vi "module.vi"(6 "cmd channel":T2) -> (7 "response":T2)   [LabVIEW 2023, in "Camera Calibration.lvlib"]
uses:
  Camera Calibration.lvlib
  <extravilib>/ChannelInstances/Messenger-t'Message Queue.lvlib-Message Cluster.ctl'/))Channel.ctl
  <vilib>/DLR/CMH Library/Message Queue/Message Cluster.ctl
  <vilib>/DLR/Graphs/Detail Graph/Detail Graph.lvclass
  C:/Program Files/National Instruments/LabVIEW 2023/vi.lib/DLR/Graphs/Base Graph/Base Graph.lvclass
  <vilib>/Utility/miscctls.llb/LVPoint32TypeDef.ctl
  <vilib>/DLR/CMH Library/Message Queue/Enqueue Message.vi
  c1bcd614-dbd8-4c7e-9590-75ab6b9c2f97.vi
  5a16af59-63b5-408a-9197-58993c91bf3e.vi
  e40aba5b-5f5a-4406-9bae-245098e35ac7.vi
  702dd1aa-c489-4f6b-9c67-8e13a44c3bd1.vi
  480c1a3a-5302-4998-8e9b-bb535253195f.vi
  <extravilib>/ChannelInstances/Messenger-t'Message Queue.lvlib-Message Cluster.ctl'/Write With Abort.vi
  <extravilib>/ChannelInstances/Event Messenger-bool/Instantiate.vi
  <extravilib>/ChannelInstances/Event Messenger-bool/))Channel.vi
  <extravilib>/ChannelInstances/Messenger-t'Message Queue.lvlib-Message Cluster.ctl'/Endpoint.vi
  <vilib>/Utility/inputDevices.llb/keyboardAcquire.vi
  <vilib>/Utility/error.llb/Error Cluster From Error Code.vi
  <vilib>/ErrorRing/Error Ring.xnode
  <vilib>/DLR/CMH Library/Message Queue.lvlib
  <vilib>/DLR/CMH Library/Message Queue Helper.lvlib
  <extravilib>/ChannelInstances/Event Messenger-bool.lvlib
  <vilib>/DLR/Graphs/Base Graph/Base Graph.lvclass
  OpenCV-Calibration-LabVIEW-Wrapper/build/x64/Debug/OpenCV-Calibration-LabVIEW-Wrapper.dll
  C:/Program Files/National Instruments/LabVIEW 2023/vi.lib/DLR/Graphs/Detail Graph/Detail Graph.lvclass
  <extravilib>/ChannelInstances/Messenger-t'Message Queue.lvlib-Message Cluster.ctl'.lvlib
panel:
  in  "Main Control":enum32{"Feature Extraction", "Empty"}(tab)
  out "Selection Mask":T1 {"Polygon"."Y [px]" format="%#_5g"}
  out "Extracted Points":cluster{"X [px]":sgl, "Y [px]":sgl}[](array[cluster]) {"Y [px]" format="%#_5g"; "X [px]" format="%#_5g"}
  in  "Extract Corners":bool
  out "Intensity Width Graph":cluster{"Array":dbl[], "Array":dbl[]}(graph)
  out "Signal Map":u16[][](graph)
  out "Intensity Height Graph":cluster{"Array":dbl[], "Array":dbl[]}(graph)
  in  "Image #":u16
  in  "Close Button":bool
  out "Log":string
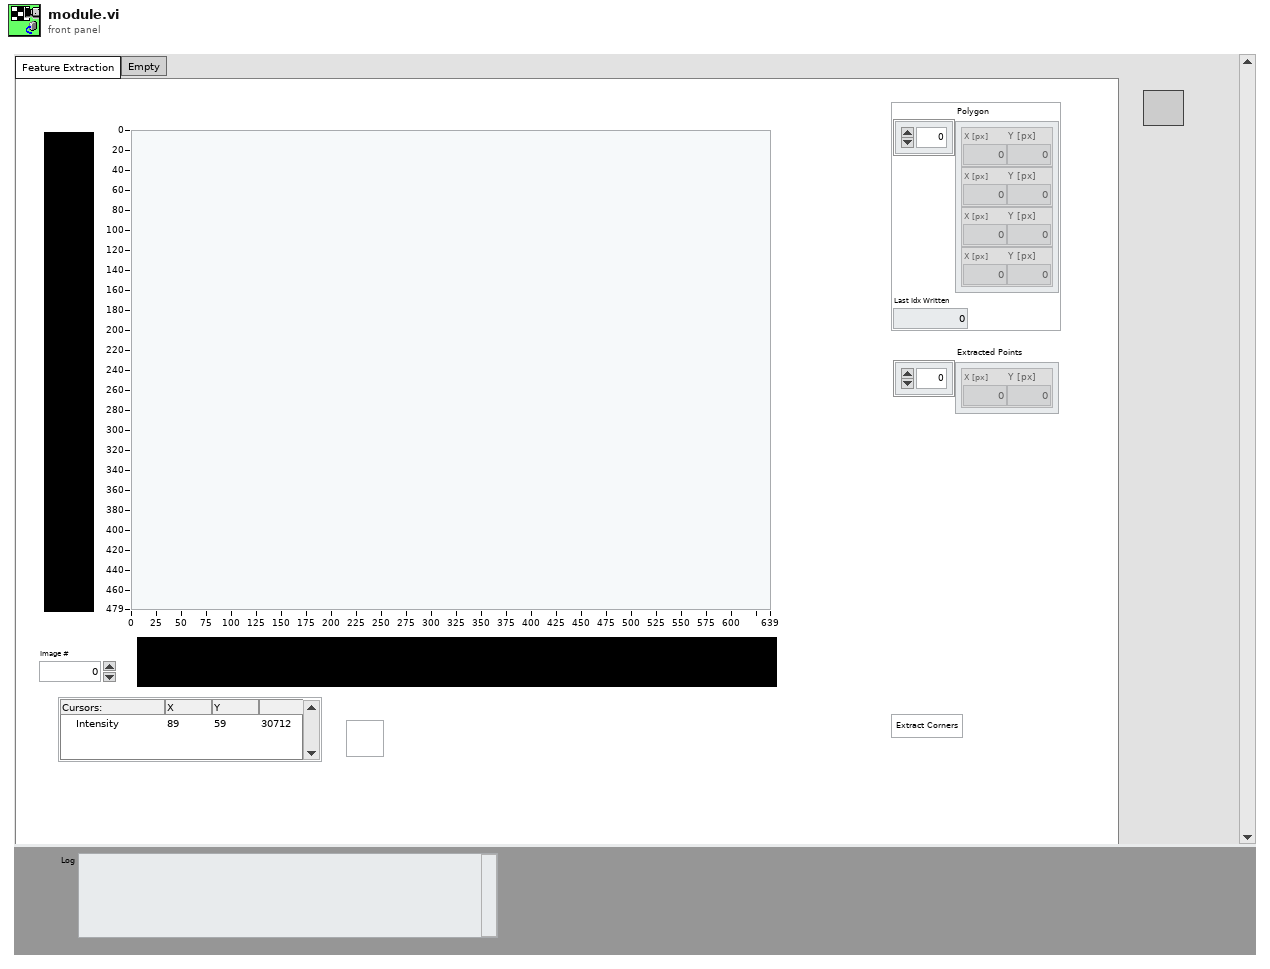
[diagram p1: front panel]
types:
  T1 = cluster{"Polygon":cluster{"X [px]":i32, "Y [px]":dbl}[], "Last Idx Written":i32}
  T2 = typedef "Messenger-t'Message Queue.lvlib-Message Cluster.ctl'.lvlib/))Channel.ctl" = refnum<queue>
  T3 = cluster{"Images":u16[][][], "Overlays":picture[], "Masks Array":cluster{"Polygon":cluster{"X [px]":i32, "Y [px]":i32}[], "Last Idx Written":i32}[], "Idx":i32, "Extracted Points":cluster{"X [px]":sgl, "Y [px]":sgl}[][]}
  T4 = typedef "LVPoint32TypeDef.ctl" = cluster{"Horizontal":i32, "Vertical":i32}
  T5 = enum16{"0", "1", "2", "3", "4", "5", "6", "7", "8", "9", "A", "B", "C", "D", "E", "F", "G", "H", "I", "J", "K", "L", "M", "N", "O", "P", "Q", "R", "S", "T", "U", "V", "W", "X", "Y", "Z", "F1", "F2", "F3", "F4", "F5", "F6", "F7", "F8", "F9", "F10", "F11", "F12", "F13", "F14", "F15", "ADD", "BACK", "BACKSLASH", "CAPITAL", "COMMA", "DECIMAL", "DELETE", "DIVIDE", "DOWN", "END", "EQUALS", "ESCAPE", "GRAVE (`)", "HOME", "INSERT", "LBRACKET", "LCONTROL", "LEFT", "L ALT", "LSHIFT", "LWIN", "MINUS", "MULTIPLY", "NEXT", "NUMLOCK", "NUMPAD_0", "NUMPAD_1", "NUMPAD_2", "NUMPAD_3", "NUMPAD_4", "NUMPAD_5", "NUMPAD_6", "NUMPAD_7", "NUMPAD_8", "NUMPAD_9", "PAUSE", "PERIOD", "PRIOR (PG UP)", "RBRACKET", "RCONTROL", "RETURN", "RIGHT", "R ALT", "RSHIFT", "RWIN", "SCROLL", "SEMICOLON", "SLASH", "SPACE", "SUBTRACT", "TAB", "UP", "ENTER (num pad)", "' (quote)"}[]
  T6 = enum16{"0", "1", "2", "3", "4", "5", "6", "7", "8", "9", "A", "B", "C", "D", "E", "F", "G", "H", "I", "J", "K", "L", "M", "N", "O", "P", "Q", "R", "S", "T", "U", "V", "W", "X", "Y", "Z", "F1", "F2", "F3", "F4", "F5", "F6", "F7", "F8", "F9", "F10", "F11", "F12", "F13", "F14", "F15", "ADD", "BACK", "BACKSLASH", "CAPITAL", "COMMA", "DECIMAL", "DELETE", "DIVIDE", "DOWN", "END", "EQUALS", "ESCAPE", "GRAVE (`)", "HOME", "INSERT", "LBRACKET", "LCONTROL", "LEFT", "L ALT", "LSHIFT", "LWIN", "MINUS", "MULTIPLY", "NEXT", "NUMLOCK", "NUMPAD_0", "NUMPAD_1", "NUMPAD_2", "NUMPAD_3", "NUMPAD_4", "NUMPAD_5", "NUMPAD_6", "NUMPAD_7", "NUMPAD_8", "NUMPAD_9", "PAUSE", "PERIOD", "PRIOR (PG UP)", "RBRACKET", "RCONTROL", "RETURN", "RIGHT", "R ALT", "RSHIFT", "RWIN", "SCROLL", "SEMICOLON", "SLASH", "SPACE", "SUBTRACT", "TAB", "UP", "ENTER (num pad)", "' (quote)"}
  T7 = cluster{"Polygon":cluster{"X [px]":dbl, "Y [px]":dbl}[], "Last Idx Written":i32}
  T8 = cluster{"IntGraph Ref":refnum<vi>, "Y-Graph Ref":refnum<vi>, "X-Graph Ref":refnum<vi>}
  T9 = cluster{"Polygon":cluster{"X":dbl, "Y":dbl}[], "Last Idx Written":i32}
  T10 = cluster{"Polygon":cluster{"X [px]":i32, "Y [px]":i32}[], "Last Idx Written":i32}[]
  T11 = cluster{"Polygon":cluster{"X [px]":i32, "Y [px]":i32}[], "Last Idx Written":i32}
  T12 = cluster{"Polygon":cluster{"X [px]":dbl, "Y [px]":dbl}[], "Last Idx Written":i32}[]
  T13 = typedef "Event Messenger-bool.lvlib/))Channel.ctl" = refnum<queue>
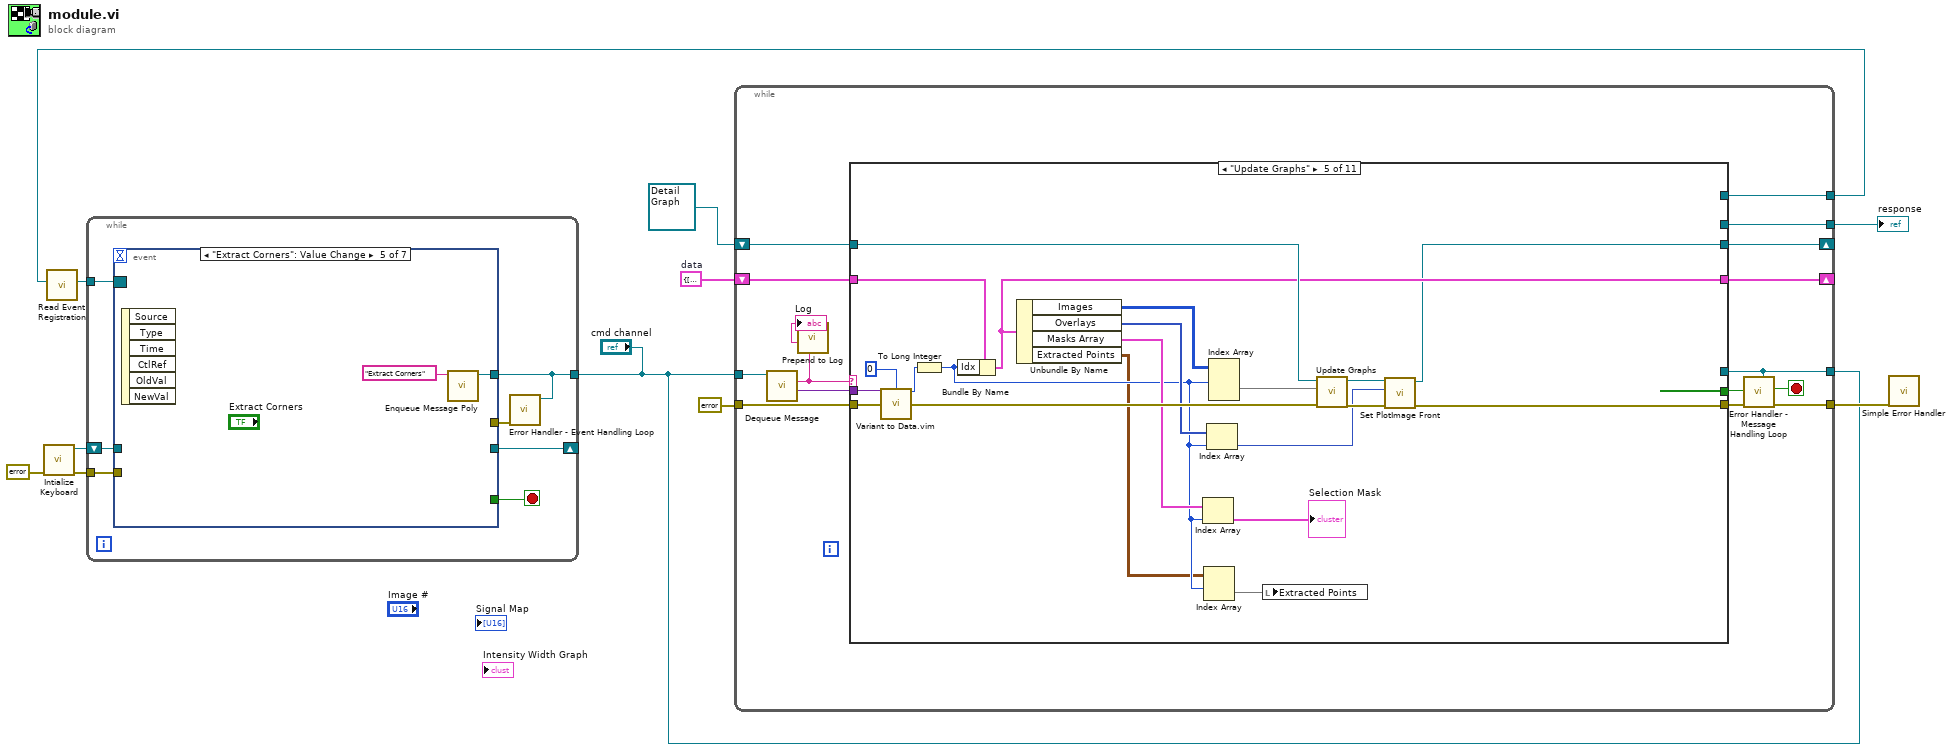
[diagram p0: block diagram]
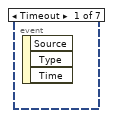
[diagram p2: hidden frame]
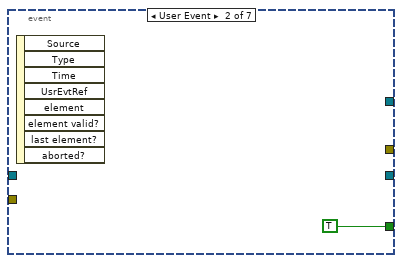
[diagram p3: hidden frame]
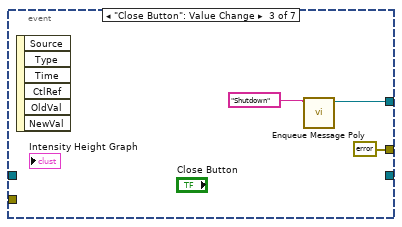
[diagram p4: hidden frame]
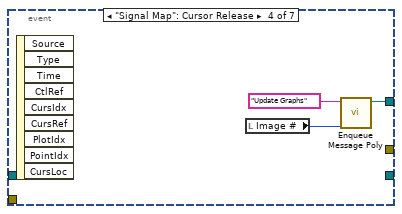
[diagram p5: hidden frame]
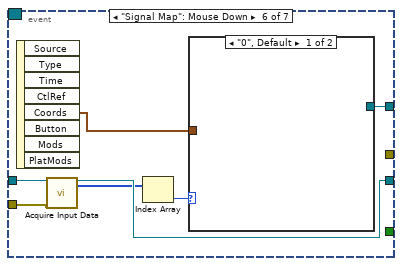
[diagram p6: hidden frame]
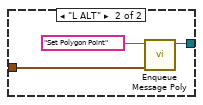
[diagram p7: hidden frame]
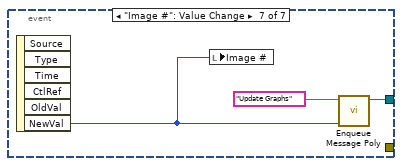
[diagram p8: hidden frame]
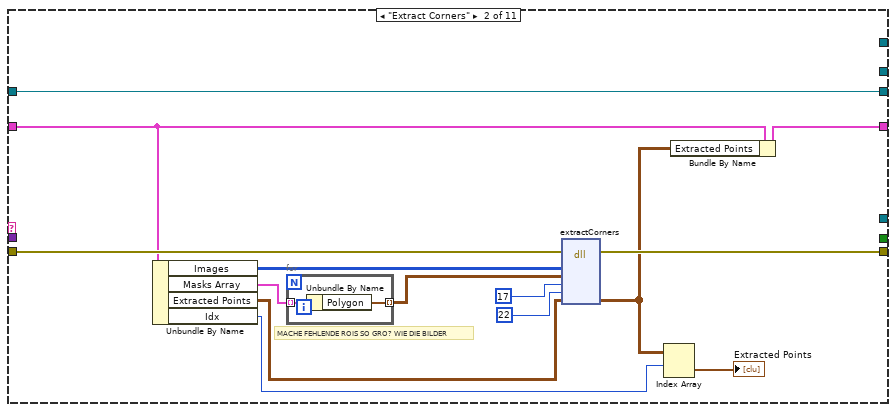
[diagram p10: hidden frame]
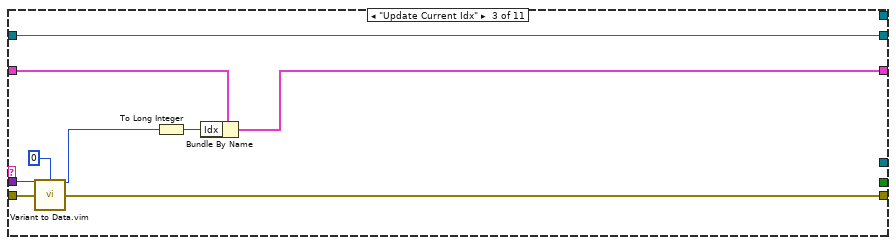
[diagram p11: hidden frame]
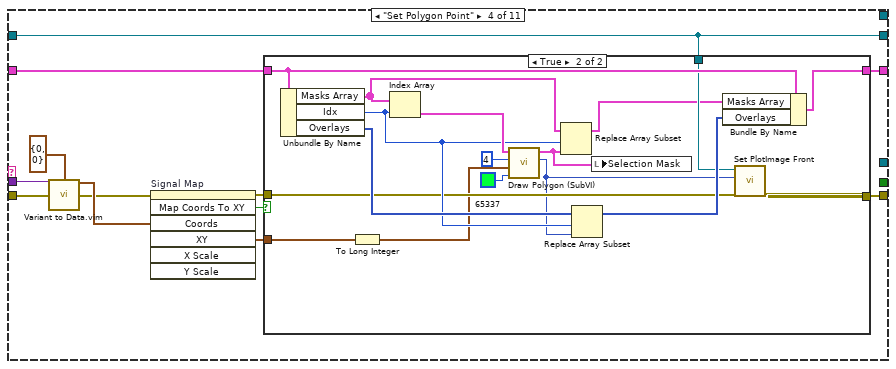
[diagram p12: hidden frame]
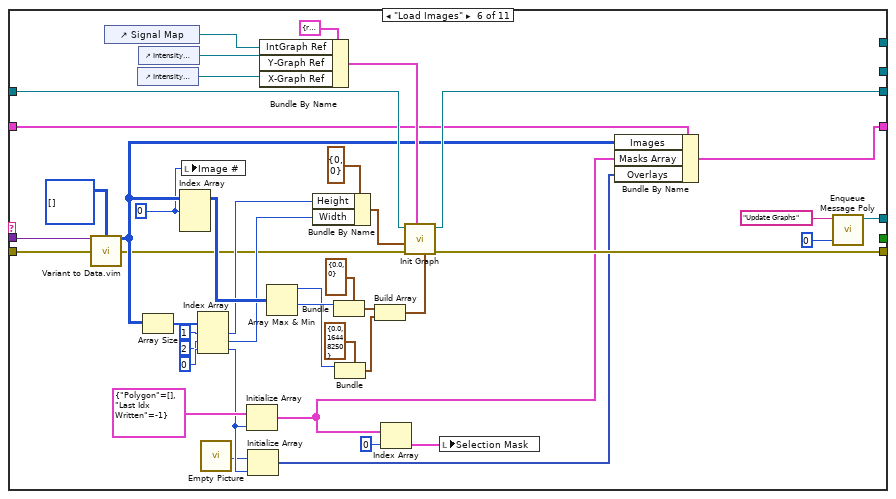
[diagram p14: hidden frame]
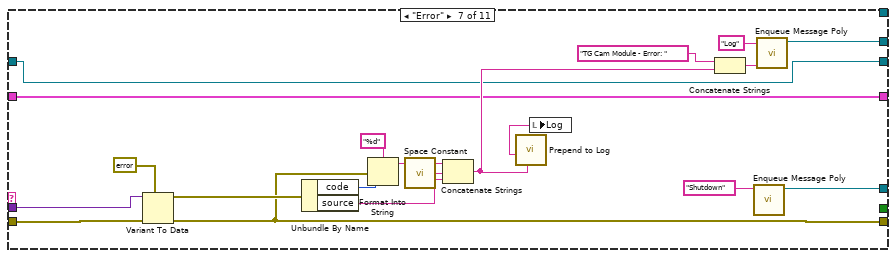
[diagram p15: hidden frame]
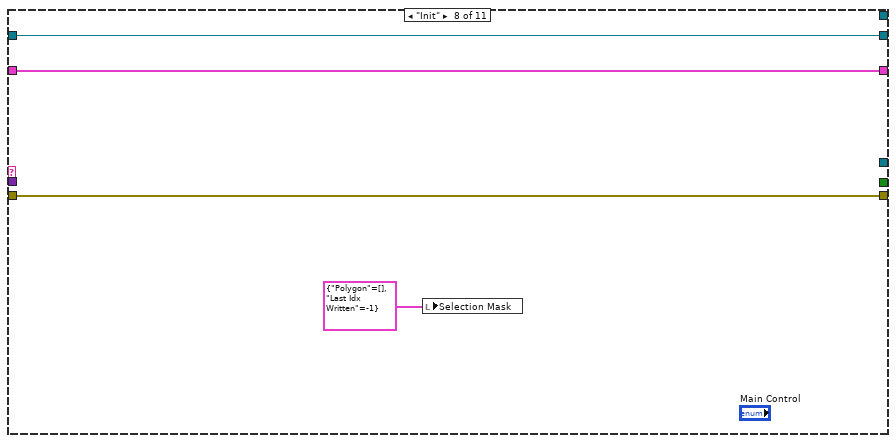
[diagram p16: hidden frame]
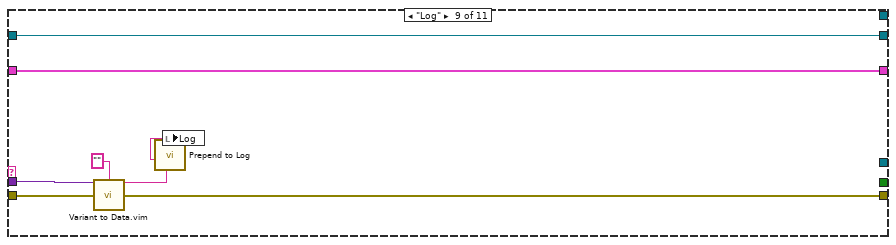
[diagram p17: hidden frame]
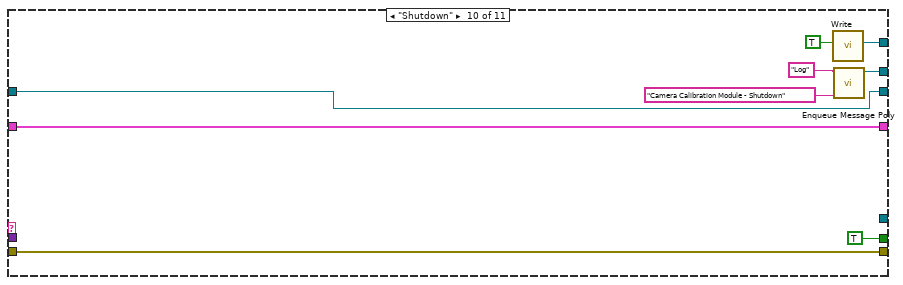
[diagram p18: hidden frame]
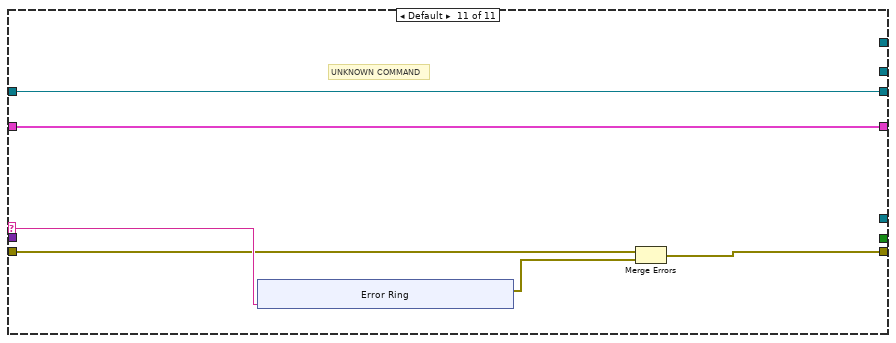
[diagram p19: hidden frame]
diagram:
  w1 = T3 {"Images"=[], "Overlays"=[], "Masks Array"=[], "Idx"=0, "Extracted Points"=[]}  # data
  n1 = call <vilib>:"Intialize Keyboard.vi"("error in (no error)"=errorcluster {"status"=FALSE, "code"=0, "source"=""}) -> ("error out"=w3:errorcluster, "device ID"=w2:refnum<k1>)  [unwired: 9 in]
  n2 = call <extravilib>:"Read Event Registration.vi"("channel"=w10) -> ("event registration refnum"=w9:refnum<event-registration>)  [unwired: 10 in]
  n3 = while {
    tunnel: [w15] -> w6
    tunnel: w9 -> [w17]
    tunnel: w3 -> [w14]
    shift-right: [w12] -> _
    shift-left: w2 -> [w13]
    stop <- w18 stop-if-true
    n4 = event shown="[4] \"Extract Corners\": Value Change" {
      selector: w17 -> [_ _ _ _ _ _ _]
      dyn-events: _ -> [_ _ _ _ _ _ _]
      timeout: _ -> [_ _ _ _ _ _ _]
      tunnel: [_ _ w22 w24 w26 w29 w39] -> w15
      tunnel: [_ TRUE _ _ _ _ _] -> w18
      tunnel: [_ _ errorcluster {"status"=FALSE, "code"=0, "source"=""} ("error out") _ _ _ _] -> w16
      tunnel: w14 -> [_ _ _ _ _ w34 _]
      tunnel: w13 -> [_ _ _ _ _ w33 _]
      tunnel: [_ _ _ _ _ w32 _] -> w12
      event Timeout {
        n5 = event-data() -> ()  [unwired: 1 in, 3 out]
      }
      event User Event {
        n6 = event-data() -> ()  [unwired: 1 in, 8 out]
      }
      event "Close Button": Value Change {
        n7 = event-data() -> ()  [unwired: 1 in, 6 out]
        n8 = call-poly <vilib>:"Enqueue Message Poly.vi"("Message"="Shutdown") -> ("channel"=w22:T2)  [unwired: 10 in]
      }
      event "Signal Map": Cursor Release {
        n9 = event-data() -> ()  [unwired: 1 in, 9 out]
        n10 = local read "Image #"() -> (w23:u16)
        n11 = call-poly <vilib>:"Enqueue Message Poly.vi"("Message Data"=w23, "Message"="Update Graphs") -> ("channel"=w24:T2)  [unwired: 9 in]
      }
      event "Extract Corners": Value Change {
        n12 = event-data() -> ()  [unwired: 1 in, 6 out]
        n13 = call-poly <vilib>:"Enqueue Message Poly.vi"("Message"="Extract Corners") -> ("channel"=w26:T2)  [unwired: 10 in]
      }
      event "Signal Map": Mouse Down {
        n14 = event-data() -> ("Coords"=w28:T4)  [unwired: 1 in, 7 out]
        n15 = call-poly <vilib>:"Acquire Input Data.vi"("device ID"=w33, "error in (no error)"=w34) -> ("device ID"=w32:refnum<k1>, "keys pressed"=w31:T5)  [unwired: 15 in, 1 out]
        n16 = Index Array(array=w31) -> (element=w30:T6)  [unwired: 1 in]
        n17 = case shown="\"0\", Default" w30 {
          tunnel: [_ w36] -> w29
          tunnel: w28 -> [_ w35]
          frame "0", Default {
          }
          frame "L ALT" {
            n18 = call-poly <vilib>:"Enqueue Message Poly.vi"("Message Data"=w35, "Message"="Set Polygon Point") -> ("channel"=w36:T2)  [unwired: 9 in]
          }
        }
      }
      event "Image #": Value Change {
        n19 = event-data() -> ("NewVal"=w38:u16)  [unwired: 1 in, 5 out]
        n20 = local write "Image #"(w38) -> ()
        n21 = call-poly <vilib>:"Enqueue Message Poly.vi"("Message Data"=w38, "Message"="Update Graphs") -> ("channel"=w39:T2)  [unwired: 9 in]
      }
    }
    n22 = call <vilib>:"Error Handler - Event Handling Loop.vi"("channel"=w15, "error in (no error)"=w16) -> ()  [unwired: 9 in, 1 out]
  }
  "cmd channel" <- w6
  n23 = while {
    tunnel: w6 -> [w56]
    tunnel: w6 -> [w54]
    tunnel: [w50] -> w10
    tunnel: [w48] -> w8
    tunnel: errorcluster {"status"=FALSE, "code"=0, "source"=""} ("error constant") -> [w47]
    tunnel: [w51] -> w7
    shift-right: [w41] -> _
    shift-left: w1 -> [w44]
    shift-right: [w42] -> _
    shift-left: refnum<class "Detail Graph.lvclass"> refnum ("Detail Graph out.lvclass") -> [w43]
    stop <- w52 stop-if-true
    n24 = call <vilib>:"Dequeue Message.vi"("channel"=w56) -> ("message data"=w55:variant, "message"=w49:string)  [unwired: 8 in, 1 out]
    n25 = call <vilib>:"Prepend to Log.vi"("new entry"=w49) -> ("Log out"=→"Log":string)  [unwired: 10 in]
    n26 = case shown="\"Update Graphs\"" w49 {
      selector: w49 -> [_ _ _ _ _ _ _ _ _ _ w223]
      tunnel: w55 -> [_ _ w81 w94 w132 w176 w190 _ w207 _ _]
      tunnel: w47 -> [w59 w73 w84 w96 w136 w178 w193 w202 w210 w218 w222]
      tunnel: [_ _ _ _ _ _ _ _ _ TRUE _] -> w53
      tunnel: [_ _ _ _ _ w157 w188 _ _ _ _] -> w54
      tunnel: [w59 w71 w82 w88 w123 w171 w189 w202 w209 w218 w225] -> w46
      tunnel: [_ _ _ _ _ _ _ _ _ w216 _] -> w50
      tunnel: [_ _ _ _ _ _ w184 _ _ w214 _] -> w48
      tunnel: w44 -> [w57 w70 w79 w86 w130 w148 w179 w200 w203 w211 w220]
      tunnel: w43 -> [w58 w72 w83 w87 w135 w173 w180 w201 w204 w212 w221]
      tunnel: [w58 w72 w83 w87 w122 w172 w180 w201 w204 w212 w221] -> w42
      tunnel: [w57 w63 w76 w85 w128 w144 w179 w200 w203 w211 w220] -> w41
      frame "DUPLICATE THIS CASE" {
      }
      frame "Extract Corners" {
        # "MACHE FEHLENDE ROIS SO GRO? WIE DIE BILDER"
        n27 = Unbundle By Name(w70) -> ("Images"=w69:u16[][][], "Masks Array"=w68:T10, "Extracted Points"=w66:cluster{"X [px]":sgl, "Y [px]":sgl}[][], "Idx"=w65:i32)
        n28 = for {
          tunnel: w68 -> [w75] mode=indexing
          tunnel: [w74] -> w67 mode=indexing
          n29 = Unbundle By Name(w75) -> ("Polygon"=w74:cluster{"X [px]":i32, "Y [px]":i32}[])
        }
        n30 = dll-call lib="D:/git/Camera-Calibration-LabVIEW/OpenCV-Calibration-LabVIEW-Wrapper/build/x64/Debug/OpenCV-Calibration-LabVIEW-Wrapper.dll" fn="extractCorners"(error in=w73, "images"=w69, "maskPolygons"=w67, "cbRows"=17, "cbCols"=22, "extractedPoints"=w66) -> (error out=w71:errorcluster, "extractedPoints"=w62:cluster{"X [px]":sgl, "Y [px]":sgl}[][])  [unwired: 7 in, 1 out]
        n31 = Index Array(array=w62, index (row)=w65) -> (element=→"Extracted Points":cluster{"X [px]":sgl, "Y [px]":sgl}[])  [unwired: 1 in]
        n32 = Bundle By Name(cluster=w70, "Extracted Points"=w62) -> (w63:T3)
      }
      frame "Update Current Idx" {
        n33 = call "Variant to Data.vim"("variant"=w81, "type"=u16 0, "Error In"=w84) -> ("data"=w77:u16, "Error Out"=w82:errorcluster)  [unwired: 11 in]
        n34 = To Long Integer(number=w77) -> (32bit integer=w78:i32)
        n35 = Bundle By Name(cluster=w79, "Idx"=w78) -> (w76:T3)
      }
      frame "Set Polygon Point" {
        n36 = call "Variant to Data.vim"("variant"=w94, "type"=T4 {"Horizontal"=0, "Vertical"=0} ("Coords"), "Error In"=w96) -> ("data"=w93:T4, "Error Out"=w89:errorcluster)  [unwired: 11 in]
        n37 = invoke on="Signal Map" class="IntGraph (strict)" method="Map Coords To XY"(error in=w89, "Coords"=w93) -> (error out=w90:errorcluster, "Map Coords To XY"=w91:bool, "XY"=w92:cluster{"X":dbl, "Y":dbl})  [unwired: 5 in, 4 out]
        n38 = case shown="True" w91 {
          tunnel: w92 -> [_ w114]
          tunnel: w90 -> [w98 w106]
          tunnel: [w98 w105] -> w88
          tunnel: w87 -> [_ w104]
          tunnel: w86 -> [w97 w111]
          tunnel: [w97 w112] -> w85
          frame False {
          }
          frame True {
            n39 = Unbundle By Name(w111) -> ("Masks Array"=w100:T10, "Idx"=w108:i32, "Overlays"=w109:picture[])
            n40 = To Long Integer(number=w114) -> (32bit integer=w102:cluster{"X":i32, "Y":i32})
            n41 = Index Array(array=w100, index=w108) -> (element=w110:T11)
            n42 = call "Draw Polygon (SubVI).vi"("color)"=u32 65337, "New Point"=w102, "Nbr Polygon Points"=4, "Selection Mask in"=w110) -> ("new picture"=w103:picture, "Selection Mask out"=w99:T11)  [unwired: 6 in]
            n43 = Replace Array Subset(array=w100, new element=w99, index=w108) -> (w101:T10)
            n44 = Replace Array Subset(array=w109, new element=w103, index=w108) -> (w107:picture[])
            n45 = local write "Selection Mask"(w99) -> ()
            n46 = Bundle By Name(cluster=w111, "Masks Array"=w101, "Overlays"=w107) -> (w112:T3)
            n47 = call <vilib>:"Set PlotImage Front.vi"("error in (no error)"=w106, "Plot Images:Front"=w103, "Base Graph in"=w104) -> ("error out"=w105:errorcluster)  [unwired: 7 in, 1 out]
          }
        }
      }
      frame "Update Graphs" {
        n48 = call "Variant to Data.vim"("variant"=w132, "type"=u16 0, "Error In"=w136) -> ("data"=w129:u16, "Error Out"=w127:errorcluster)  [unwired: 11 in]
        n49 = To Long Integer(number=w129) -> (32bit integer=w117:i32)
        n50 = Bundle By Name(cluster=w130, "Idx"=w117) -> (w128:T3)
        n51 = Unbundle By Name(w128) -> ("Images"=w133:u16[][][], "Overlays"=w126:picture[], "Masks Array"=w120:T10, "Extracted Points"=w116:cluster{"X [px]":sgl, "Y [px]":sgl}[][])
        n52 = Index Array(array=w120, index=w117) -> (element=→"Selection Mask":T11)
        n53 = Index Array(array=w116, index (row)=w117) -> (element=w118:cluster{"X [px]":sgl, "Y [px]":sgl}[])  [unwired: 1 in]
        n54 = Index Array(array=w126, index=w117) -> (element=w121:picture)
        n55 = Index Array(array=w133, index (dim 0)=w117) -> (element=w134:u16[][])  [unwired: 2 in]
        n56 = local write "Extracted Points"(w118) -> ()
        n57 = call <vilib>:"Update Graphs.vi"("error in (no error)"=w127, "image"=w134, "Detail Graph in"=w135) -> ("error out"=w124:errorcluster, "Detail Graph out"=w125:refnum<class "Detail Graph.lvclass">)  [unwired: 6 in, 1 out]
        n58 = call <vilib>:"Set PlotImage Front.vi"("error in (no error)"=w124, "Plot Images:Front"=w121, "Base Graph in"=w125) -> ("error out"=w123:errorcluster, "Base Graph out"=w122:refnum<class "Detail Graph.lvclass">)  [unwired: 7 in]
      }
      frame "Load Images" {
        w143 = 0 ("index (page)")
        n59 = call "Variant to Data.vim"("variant"=w176, "type"=u16[][][] [], "Error In"=w178) -> ("data"=w147:u16[][][], "Error Out"=w137:errorcluster)  [unwired: 11 in]
        n60 = control-ref of="Signal Map"() -> (w168:refnum<vi>)
        n61 = control-ref of="Intensity Width Graph"() -> (w167:refnum<vi>)
        n62 = control-ref of="Intensity Height Graph"() -> (w169:refnum<vi>)
        n63 = Array Size(array=w147) -> (size(s)=w155:i32[])
        n64 = Index Array(array=w147, index (dim 0)=w143) -> (element=w165:u16[][])  [unwired: 2 in]
        n65 = local write "Image #"(w143) -> ()
        n66 = Index Array(array=w155, index #1=1 ("index"), index #2=2 ("index"), index #3=0 ("index")) -> (element #1=w150:i32, element #2=w149:i32, element #3=w142:i32)
        n67 = call "Empty Picture"() -> ("empty picture"=w141:picture)
        n68 = Initialize Array(T7 {"Polygon"=[], "Last Idx Written"=-1} ("Selection Mask"), w142) -> (w145:T12)
        n69 = Initialize Array(w141, w142) -> (w140:picture[])
        n70 = Bundle By Name(cluster=T8 {"IntGraph Ref"=refnum, "Y-Graph Ref"=refnum, "X-Graph Ref"=refnum} ("Graphs"), "IntGraph Ref"=w168, "Y-Graph Ref"=w169, "X-Graph Ref"=w167) -> (w166:T8)
        n71 = Array Max & Min(array=w165) -> (max value=w160:u16, min value=w163:u16)  [unwired: 2 out]
        n72 = Bundle By Name(cluster=cluster{"Height":u32, "Width":u32} {"Height"=0, "Width"=0} ("Images Size"), "Height"=w150, "Width"=w149) -> (w175:cluster{"Height":u32, "Width":u32})
        n73 = Bundle(cluster=cluster{"Numeric":dbl, "Numeric":u32} {"Numeric"=0.0, "Numeric"=0} ("Cluster"), "Numeric"=w163) -> (w162:cluster{"Numeric":dbl, "Numeric":u32})  [unwired: 1 in]
        n74 = Bundle(cluster=cluster{"Numeric":dbl, "Numeric":u32} {"Numeric"=0.0, "Numeric"=16448250} ("Cluster"), "Numeric"=w160) -> (w159:cluster{"Numeric":dbl, "Numeric":u32})  [unwired: 1 in]
        n75 = Build Array(w162, w159) -> (w158:cluster{"Numeric":dbl, "Numeric":u32}[])
        n76 = Index Array(array=w145, index=0) -> (element=w138:T7)
        n77 = call <vilib>:"Init Graph.vi"("Z Scale.Marker Values[]"=w158, "Graphs"=w166, "error in (no error)"=w137, "Images Size"=w175, "Detail Graph.lvclass"=w173) -> ("error out"=w171:errorcluster, "Detail Graph out.lvclass"=w172:refnum<class "Detail Graph.lvclass">)  [unwired: 5 in]
        n78 = local write "Selection Mask"(w138) -> ()
        n79 = Bundle By Name(cluster=w148, "Images"=w147, "Masks Array"=w145, "Overlays"=w140) -> (w144:T3)
        n80 = call-poly <vilib>:"Enqueue Message Poly.vi"("Message Data"=0 ("index (page)"), "Message"="Update Graphs") -> ("channel"=w157:T2)  [unwired: 9 in]
      }
      frame "Error" {
        n81 = Variant To Data(error in=w193, type=errorcluster {"status"=FALSE, "code"=0, "source"=""} ("error in (no error)"), Variant=w190) -> (data=w192:errorcluster, error out=w189:errorcluster)
        n82 = Unbundle By Name(w192) -> ("code"=w198:i32, "source"=w195:string)
        n83 = Format Into String(format string="%d", error in=w189, w198) -> (resulting string=w197:string)  [unwired: 1 in, 1 out]
        n84 = call <vilib>:"Space Constant.vi"() -> ("String"=w196:string)
        n85 = Concatenate Strings(w197, w196, w195) -> (w181:string)
        n86 = call <vilib>:"Prepend to Log.vi"("new entry"=w181) -> ("Log out"=w182:string)  [unwired: 10 in]
        n87 = local write "Log"(w182) -> ()
        n88 = Concatenate Strings("TG Cam Module - Error: " ("Message"), w181) -> (w183:string)
        n89 = call-poly <vilib>:"Enqueue Message Poly.vi"("Message"="Shutdown") -> ("channel"=w188:T2)  [unwired: 10 in]
        n90 = call-poly <vilib>:"Enqueue Message Poly.vi"("Message Data"=w183, "Message"="Log") -> ("channel"=w184:T2)  [unwired: 9 in]
      }
      frame "Init" {
        n91 = local write "Selection Mask"(T9 {"Polygon"=[], "Last Idx Written"=-1} ("Selection Mask")) -> ()
      }
      frame "Log" {
        n92 = call "Variant to Data.vim"("variant"=w207, "type"="", "Error In"=w210) -> ("data"=w206:string, "Error Out"=w209:errorcluster)  [unwired: 11 in]
        n93 = call <vilib>:"Prepend to Log.vi"("new entry"=w206) -> ("Log out"=w205:string)  [unwired: 10 in]
        n94 = local write "Log"(w205) -> ()
      }
      frame "Shutdown" {
        n95 = call <extravilib>:"Write.vi"("element"=TRUE) -> ("channel"=w216:T13)  [unwired: 9 in, 1 out]
        n96 = call-poly <vilib>:"Enqueue Message Poly.vi"("Message Data"="Camera Calibration Module - Shutdown" ("Message"), "Message"="Log") -> ("channel"=w214:T2)  [unwired: 9 in]
      }
      frame Default {
        # "UNKNOWN COMMAND"
        n97 = xnode "Error Ring"("parameter 0"=w223) -> ("error out"=w224:errorcluster)
        n98 = Merge Errors(w222, w224) -> (w225:errorcluster)
      }
    }
    n99 = call <vilib>:"Error Handler - Message Handling Loop.vi"("channel"=w54, "error in (no error)"=w46, "Shutdown?"=w53) -> ("dup error in"=w51:errorcluster, "Shutdown!"=w52:bool)  [unwired: 7 in]
  }
  "response" <- w8
  n100 = call <vilib>:"Simple Error Handler.vi"("error in (no error)"=w7) -> ()  [unwired: 4 in, 5 out]
